vi "CloseMUXAllRelays.vi"(8 "error in (no error)":errorcluster, 10 "gRPCid":T2, 11 "ctet_mux in":T1) -> (0 "error out":errorcluster, 3 "ctet_mux out":T1)   [LabVIEW 2019, in "ctet_mux_User Library.lvlib"]
uses:
  ctet_mux_User Library.lvlib
  Servers/ctet_mux/gRPC lvSupport/Server API/typeDefs/grpcId.ctl
  Types/ctet_mux.ctl
  Servers/ctet_mux/ctet_mux Class/RPC Messages/measurementservice_MUXCloseAllResponse/measurementservice_MUXCloseAllResponse_Data.ctl
  Servers/ctet_mux/ctet_mux Class/RPC Messages/measurementservice_ErrorOut/measurementservice_ErrorOut_Data.ctl
  <instrlib>/niSwitch/niSwitch.llb/niSwitch Relay Action.ctl
  Types/Switch Action.ctl
  Servers/ctet_mux/ctet_mux Class/ctet_mux.lvclass
  Servers/ctet_mux/gRPC lvSupport/gprc-lvsupport.lvlib
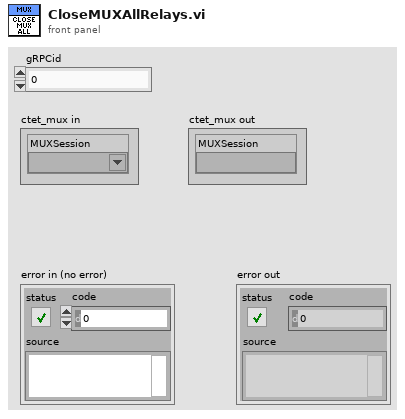
[diagram p1: front panel]
types:
  T1 = typedef "ctet_mux_User Library.lvlib/ctet_mux.ctl" = cluster{"MUXSession":refnum<k15>}
  T2 = typedef "ctet_mux.lvlib/gprc-lvsupport.lvlib/grpcId.ctl" = u64
  T3 = typedef "ctet_mux.lvlib/ctet_mux.lvclass/measurementservice_ErrorOut_Data.ctl" = cluster{"errCode":i64, "errMessage":string}
  T4 = typedef "ctet_mux.lvlib/ctet_mux.lvclass/measurementservice_MUXCloseAllResponse_Data.ctl" = cluster{"error":T3}
  T5 = typedef "ctet_mux_User Library.lvlib/Switch Action.ctl" = enum16{"Get Switch State", "Initialize", "Connect Channel", "Open Channel", "Close Relay", "Open Relay", "Disconnect/Open All"}
  T6 = typedef "niSwitch Relay Action.ctl" = i32
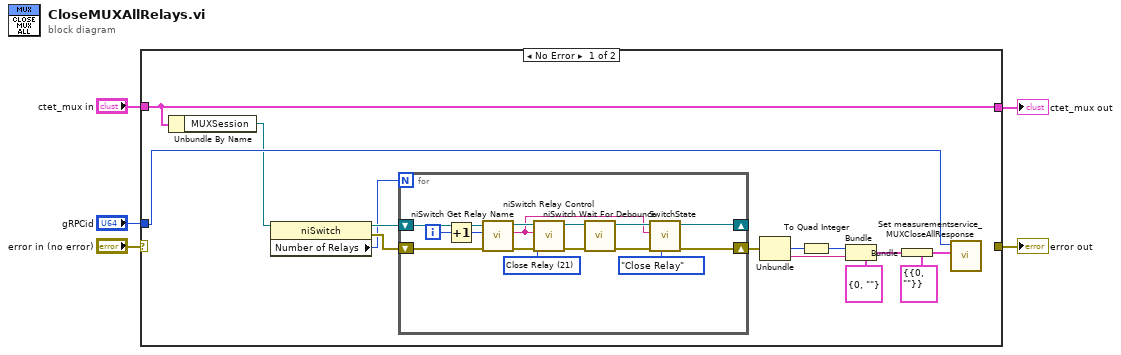
[diagram p0: block diagram]
diagram:
  n1 = case shown="No Error" "error in (no error)" {
    selector: "error in (no error)" -> [_ w36]
    tunnel: [_ w36] -> w5
    tunnel: "gRPCid" -> [w13 _]
    tunnel: "ctet_mux in" -> [w16 w35]
    tunnel: [w16 w35] -> w1
    frame No Error {
      n2 = Unbundle By Name(w16) -> ("MUXSession"=w10:refnum<k15>)
      n3 = property class="niSwitch"(reference=w10) -> (reference out=w9:refnum<k15>, error out=w8:errorcluster, "Number of Relays"=w6:i32)  [unwired: 1 in]
      n4 = for {
        N: w6 -> [_]
        shift-right: [w24] -> _
        shift-left: w9 -> [w29]
        shift-right: [w22] -> w7
        shift-left: w8 -> [w28]
        i -> [w27]
        w32 = T6 21 items=["Open Relay"=20, "Close Relay"=21] ("relay action (Close Relay)")
        n5 = Increment(x=w27) -> (x+1=w26:i32)
        n6 = call <instrlib>:"niSwitch Get Relay Name.vi"("error in (no error)"=w28, "index (1)"=w26, "instrument handle"=w29) -> ("error out"=w30:errorcluster, "relay name"=w20:string, "instrument handle out"=w31:refnum<k15>)  [unwired: 6 in]
        n7 = call <instrlib>:"niSwitch Relay Control.vi"("error in (no error)"=w30, "relay action (Close Relay)"=w32, "relay names"=w20, "instrument handle"=w31) -> ("error out"=w33:errorcluster, "instrument handle out"=w34:refnum<k15>)  [unwired: 6 in]
        n8 = call <instrlib>:"niSwitch Wait For Debounce.vi"("error in (no error)"=w33, "instrument handle"=w34) -> ("error out"=w23:errorcluster, "instrument handle out"=w25:refnum<k15>)  [unwired: 8 in]
        n9 = call "SwitchState.vi"("Switch Action"=Switch_Action."Close Relay", "error in (no error)"=w23, "channel 1"=w20, "Switch Session"=w25) -> ("error out"=w22:errorcluster, "Switch Session out"=w24:refnum<k15>)  [unwired: 5 in, 1 out]
      }
      n10 = Unbundle(w7) -> ("code"=w18:i32, "source"=w19:string)  [unwired: 1 out]
      n11 = To Quad Integer(1:w18) -> (0:w17:i64)
      n12 = Bundle(cluster=T3 {"errCode"=0, "errMessage"=""} ("error"), "errCode"=w17, "errMessage"=w19) -> (w11:T3)
      n13 = Bundle(cluster=T4 {"error"={"errCode"=0, "errMessage"=""}} ("measurementservice_MUXCloseAllResponse_Data"), "error"=w11) -> (w14:T4)
      n14 = call "Set measurementservice_MUXCloseAllResponse.vi"("Message Data"=w14, "gRPCid"=w13) -> ()  [unwired: 9 in, 1 out]
    }
    frame Error {
    }
  }
  "error out" <- w5
  "ctet_mux out" <- w1
